vi "pcfs_cleanup_queues.vi"(8 "error in (no error)":errorcluster, 11 "pcfs in":refnum<class "pcfs.lvclass">) -> (0 "error out":errorcluster, 3 "pcfs out":refnum<class "pcfs.lvclass">)   [LabVIEW 2015, in "pcfs.lvclass"]
uses:
  pcfs.lvclass
  pcfs.lvclass/pcfs.ctl
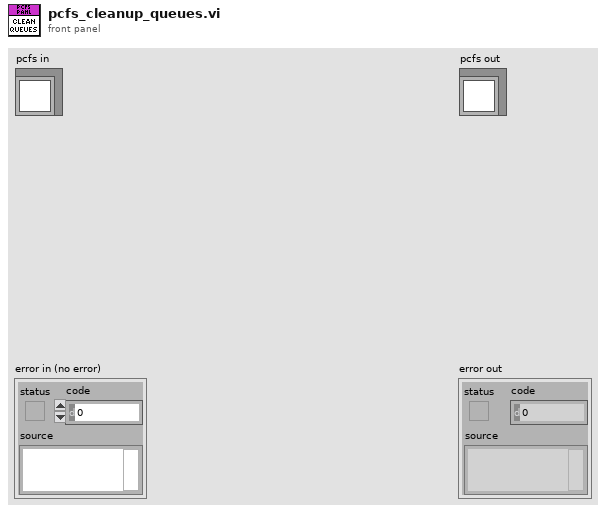
[diagram p1: front panel]
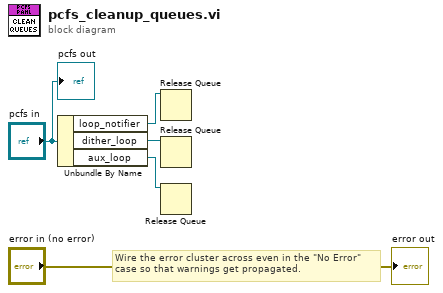
[diagram p0: block diagram]
diagram:
  # "Wire the error cluster across even in the \"No Error\"\ncase so that warnings get propagated."
  n1 = Unbundle By Name("pcfs in") -> ("loop_notifier"=w3:refnum<queue>, "dither_loop"=w2:refnum<queue>, "aux_loop"=w1:refnum<queue>)
  n2 = Release Queue(queue=w3) -> ()  [unwired: 2 in, 3 out]
  n3 = Release Queue(queue=w2) -> ()  [unwired: 2 in, 3 out]
  n4 = Release Queue(queue=w1) -> ()  [unwired: 2 in, 3 out]
  "error out" <- "error in (no error)"
  "pcfs out" <- "pcfs in"
